vi "Set_Parameter_Instrument (Json).vi"(8 "error in (no error)":errorcluster caption="entrée d'erreur (pas d'erreur)", 10 "Parameter (Json)":string, 11 "Show_Information en entrée":refnum<class "Wait_CloseFixture.lvclass">) -> (0 "error out":errorcluster caption="sortie d'erreur", 3 "Show_Information en sortie":refnum<class "Wait_CloseFixture.lvclass">)   [LabVIEW 2020, in "Library Test.lvlib" / "Wait_CloseFixture.lvclass"]
uses:
  Wait_CloseFixture.lvclass
  C:/Users/ngarcin/OneDrive - Altyor/Standard TB/Class/Test/Test (Default)/Test (Default).lvclass
  Commun VI/TypeDef/Commande DIO/Parameter DIO.ctl
  DIO/Class DIO (Default)/Class DIO (Default).lvclass
  Wait_CloseFixture.lvclass/Wait_CloseFixture.ctl
  JSON API/JSON Value/Set from JSON string.vi
  JSON API/Variant JSON/Variant to JSON.vi
  JSON API/JSON Value/Get Item by name array.vi
  Test_Without_Instr/Test_Without_Inst.lvclass
  Instrument/Instrument (Default)/Class Instrument (Default).lvclass
  JSON API/JSON Value/JSON Value.lvclass
  JSON API/Variant JSON/Variant JSON.lvlib
  JSON API/Get Polymorphic/JSON GetSet.lvlib
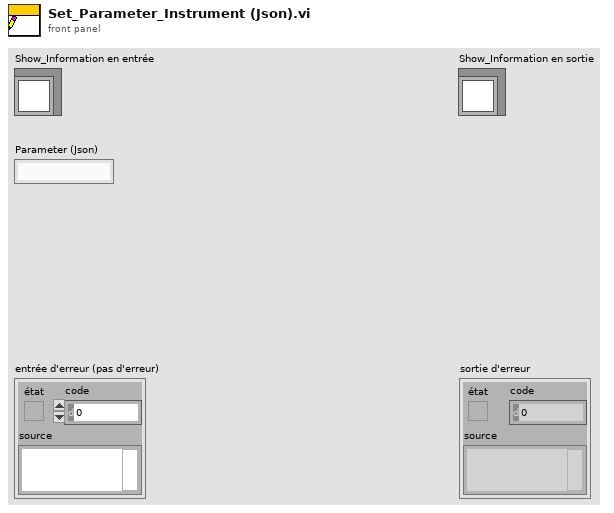
[diagram p1: front panel]
types:
  T1 = cluster{"Information_Operator":string, "Path_Picture":path, "Timeout (ms)":u64, "Function":enum16{"Write", "Read"}, "Line":u8, "Port":u8}
  T2 = typedef "Parameter DIO.ctl" = cluster{"Device_Com_Port":string, "Port":u8, "Line":u8, "Function":enum16{"Write", "Read"}, "Class DIO":refnum<class "Class DIO (Default).lvclass">}
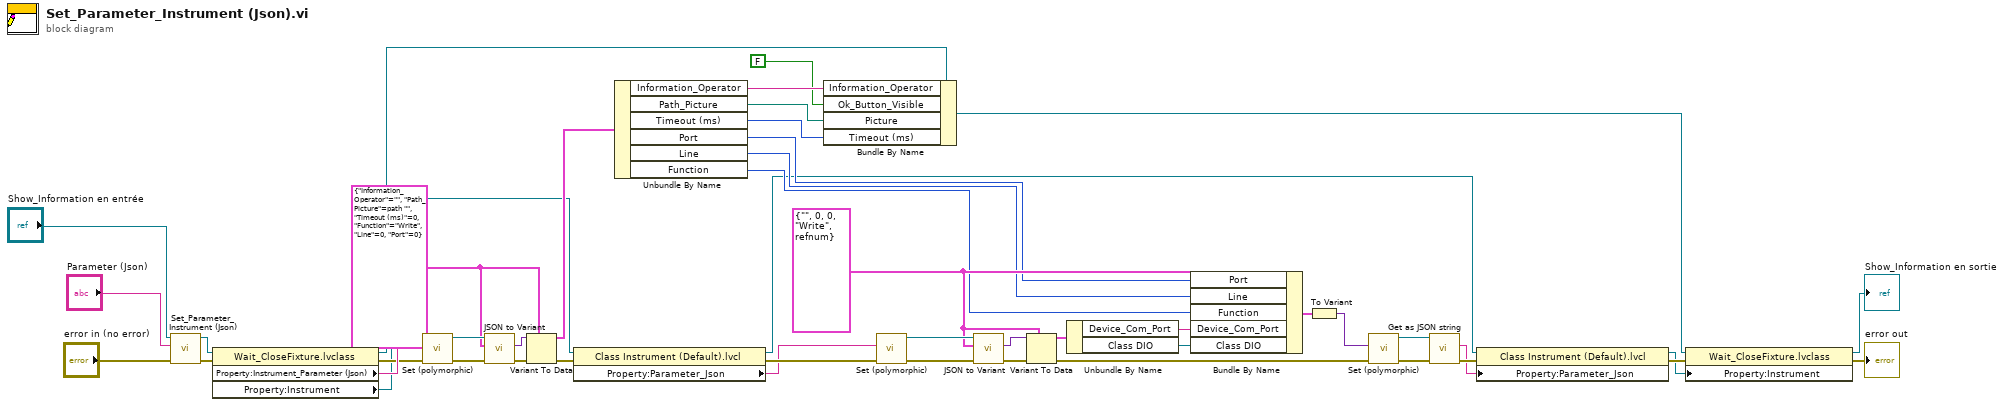
[diagram p0: block diagram]
diagram:
  w14 = T1 {"Information_Operator"="", "Path_Picture"=path "", "Timeout (ms)"=0, "Function"=enum."Write", "Line"=0, "Port"=0} ("Cluster des données privées de classe")
  w20 = T2 {"Device_Com_Port"="", "Port"=0, "Line"=0, "Function"=enum."Write", "Class DIO"=refnum} ("Parameter")
  n1 = call-parent "Set_Parameter_Instrument (Json).vi"("error in (no error)"="error in (no error)", "Parameter (Json)"="Parameter (Json)", "Test (Default) en entrée"="Show_Information en entrée") -> ("error out"=w36:errorcluster, "Test (Default) en sortie"=w37:refnum<class "Wait_CloseFixture.lvclass">)  [unwired: 7 in]
  n2 = property class="Wait_CloseFixture.lvclass"(reference=w37, error in=w36) -> (reference out=w35:refnum<class "Wait_CloseFixture.lvclass">, error out=w42:errorcluster, "Property:Instrument_Parameter (Json)"=w43:string, "Property:Instrument"=w13:refnum<class "Class Instrument (Default).lvclass">)
  n3 = call-poly "Set (polymorphic).vi"("error in (no error)"=w42, "JSON stream"=w43) -> ("error out"=w39:errorcluster, "JSON Value out"=w41:refnum<class "JSON Value.lvclass">)  [unwired: 7 in, 1 out]
  n4 = call "JSON to Variant.vi"("error in (no error)"=w39, "Variant (Data Type)"=w14, "JSON Value"=w41) -> ("error out"=w40:errorcluster, "Variant out"=w38:variant)  [unwired: 7 in]
  n5 = Variant To Data(error in=w40, type=w14, Variant=w38) -> (data=w34:T1, error out=w12:errorcluster)
  n6 = property class="Class Instrument (Default).lvcl"(reference=w13, error in=w12) -> (reference out=w2:refnum<class "Class Instrument (Default).lvclass">, error out=w19:errorcluster, "Property:Parameter_Json"=w15:string)
  n7 = Unbundle By Name(w34) -> ("Information_Operator"=w33:string, "Path_Picture"=w32:path, "Timeout (ms)"=w31:u64, "Port"=w11:u8, "Line"=w10:u8, "Function"=w9:enum16{"Write", "Read"})
  n8 = Bundle By Name(cluster=w35, "Information_Operator"=w33, "Ok_Button_Visible"=FALSE, "Picture"=w32, "Timeout (ms)"=w31) -> (w8:refnum<class "Wait_CloseFixture.lvclass">)
  n9 = call-poly "Set (polymorphic).vi"("error in (no error)"=w19, "JSON stream"=w15) -> ("error out"=w23:errorcluster, "JSON Value out"=w21:refnum<class "JSON Value.lvclass">)  [unwired: 7 in, 1 out]
  n10 = call "JSON to Variant.vi"("error in (no error)"=w23, "Variant (Data Type)"=w20, "JSON Value"=w21) -> ("error out"=w22:errorcluster, "Variant out"=w24:variant)  [unwired: 7 in]
  n11 = Variant To Data(error in=w22, type=w20, Variant=w24) -> (data=w17:T2, error out=w18:errorcluster)
  n12 = Unbundle By Name(w17) -> ("Device_Com_Port"=w16:string, "Class DIO"=w1:refnum<class "Class DIO (Default).lvclass">)
  n13 = Bundle By Name(cluster=w20, "Port"=w11, "Line"=w10, "Function"=w9, "Device_Com_Port"=w16, "Class DIO"=w1) -> (w26:T2)
  n14 = To Variant(anything=w26) -> (Variant=w30:variant)
  n15 = call-poly "Set (polymorphic).vi"("error in (no error)"=w18, "Variant"=w30) -> ("error out"=w28:errorcluster, "JSON Value out"=w29:refnum<class "JSON Value.lvclass">)  [unwired: 8 in]
  n16 = call "Get as JSON string.vi"("error in (no error)"=w28, "JSON Value in"=w29) -> ("error out"=w27:errorcluster, "<JSON>"=w25:string)  [unwired: 8 in]
  n17 = property class="Class Instrument (Default).lvcl"(reference=w2, error in=w27, "Property:Parameter_Json"=w25) -> (reference out=w4:refnum<class "Class Instrument (Default).lvclass">, error out=w6:errorcluster)
  n18 = property class="Wait_CloseFixture.lvclass"(reference=w8, error in=w6, "Property:Instrument"=w4) -> (reference out=→"Show_Information en sortie":refnum<class "Wait_CloseFixture.lvclass">, error out=→"error out":errorcluster)
